vi "ZCAN_AvailableTxCount.vi"(10 "CH_ID":i32, 11 "DeviceHANDLE":u32) -> (3 "return":u32)   [LabVIEW 2020, in "zlgcan.lvlib"]
uses:
  zlgcan.lvlib
  bin/zlgcan_wrap.dll
panel:
  out "error out":errorcluster
  in  "error in (no error)":errorcluster
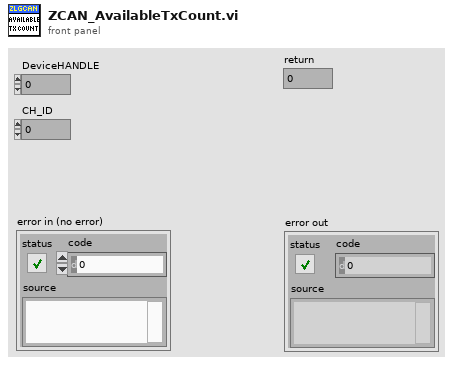
[diagram p1: front panel]
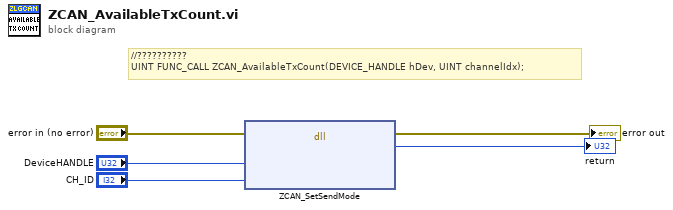
[diagram p0: block diagram]
diagram:
  # "//??????????\nUINT FUNC_CALL ZCAN_AvailableTxCount(DEVICE_HANDLE hDev, UINT channelIdx);"
  n1 = dll-call lib="D:/Git/ZLG_USBCANFD/bin/zlgcan_wrap.dll" fn="ZCAN_SetSendMode"(error in="error in (no error)", "DeviceHANDLE"="DeviceHANDLE", "CH_ID"="CH_ID") -> (error out=→"error out":errorcluster, "return"=→"return":u32)  [unwired: 4 in, 1 out]
